vi "Disabled.vi"(7 "Robot Mode":T2, 10 "Match Info":T1={"Autonomous Elapsed Seconds"=0.0, "TeleOp Elapsed Seconds"=0.0, "Disabled Elapsed Seconds"=0.0, "Visited Autonomous"=FALSE, "Visited TeleOp"=FALSE, "Visited Disabled"=FALSE, "Autonomous Settings"={"Autonomous Style"=enum."Independent", "VI Refnum"=refnum}}, 11 "Call Context":T3) -> ()   [LabVIEW 2012]
doc: "This VI is called each time a disabled packet is received from the DS. It is often used to prepare for the next robot mode, to calibrate sensors, etc."
uses:
  <vilib>/Rock Robotics/WPI/DriverStation/WPI_DriverStationDerivedRobotMode.ctl
  <vilib>/Rock Robotics/WPI/DriverStation/WPI_DriverStationRobotMode2.ctl
  <vilib>/Rock Robotics/WPI/DriverStation/WPI_DriverStationMatch Info.ctl
  Robot Global Data.vi
panel:
  out "Boolean Array 2":bool[](array[boolean])
  in  "Boolean Array":bool[](array[boolean])
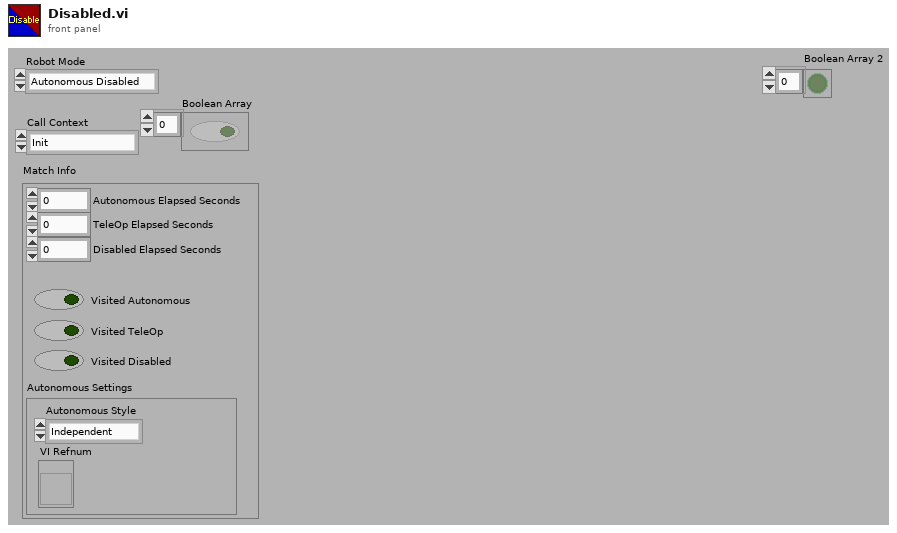
[diagram p1: front panel]
types:
  T1 = typedef "WPI_DriverStationMatch Info.ctl" = cluster{"Autonomous Elapsed Seconds":dbl, "TeleOp Elapsed Seconds":dbl, "Disabled Elapsed Seconds":dbl, "Visited Autonomous":bool, "Visited TeleOp":bool, "Visited Disabled":bool, "Autonomous Settings":cluster{"Autonomous Style":enum16{"Iterative", "Independent"}, "VI Refnum":refnum<vi>}}
  T2 = typedef "WPI_DriverStationRobotMode2.ctl" = enum16{"Autonomous Disabled", "Autonomous Enabled", "Teleop Disabled", "Teleop Enabled", "Timeout", "Finish", "Test Disabled", "Test Enabled"}
  T3 = typedef "WPI_DriverStationDerivedRobotMode.ctl" = enum16{"Init", "Execute", "Stop"}
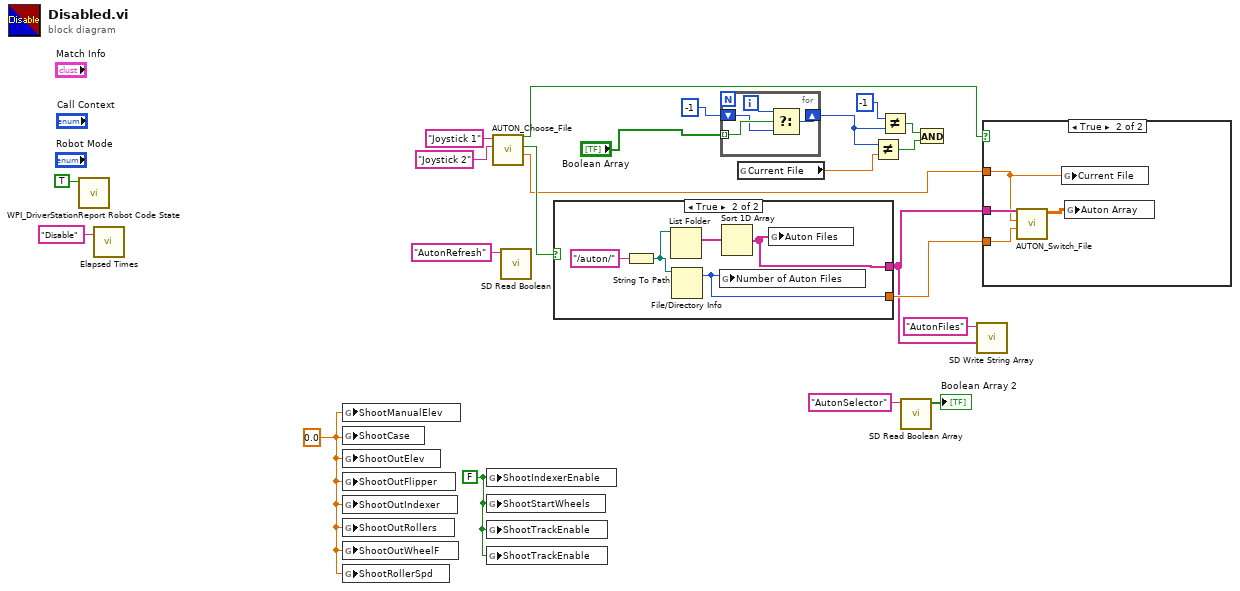
[diagram p0: block diagram]
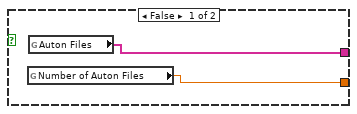
[diagram p3: hidden frame]
diagram:
  w19 = FALSE ("ShootIndexerEnable")
  w18 = 0.0 ("ShootCase")
  n1 = call <vilib>:"WPI_DriverStationReport Robot Code State.vi"("Disabled"=TRUE ("Autonomous")) -> ()  [unwired: 10 in, 1 out]
  n2 = call "Elapsed Times.vi"("Call Name"="Disable") -> ()  [unwired: 2 in, 1 out]
  n3 = global write "Robot Global Data.vi" "ShootManualElev"(w18) -> ()
  n4 = global write "Robot Global Data.vi" "ShootCase"(w18) -> ()
  n5 = global write "Robot Global Data.vi" "ShootOutElev"(w18) -> ()
  n6 = global write "Robot Global Data.vi" "ShootOutFlipper"(w18) -> ()
  n7 = global write "Robot Global Data.vi" "ShootOutIndexer"(w18) -> ()
  n8 = global write "Robot Global Data.vi" "ShootOutRollers"(w18) -> ()
  n9 = global write "Robot Global Data.vi" "ShootOutWheelF"(w18) -> ()
  n10 = global write "Robot Global Data.vi" "ShootRollerSpd"(w18) -> ()
  n11 = global write "Robot Global Data.vi" "ShootIndexerEnable"(w19) -> ()
  n12 = global write "Robot Global Data.vi" "ShootStartWheels"(w19) -> ()
  n13 = global write "Robot Global Data.vi" "ShootTrackEnable"(w19) -> ()
  n14 = global write "Robot Global Data.vi" "ShootTrackEnable"(w19) -> ()
  n15 = call "AUTON_Choose_File.vi"("Joystick 2 Refnum"="Joystick 2" ("Joystick 1 Refnum"), "Joystick 1 Refnum"="Joystick 1") -> ("Auton File"=w3:dbl, "Refresh"=w4:bool, "Allow Change"=w5:bool)  [unwired: 7 in]
  n16 = call <vilib>:"SD Read Boolean.vi"("Name"="AutonRefresh") -> ()  [unwired: 8 in, 3 out]
  n17 = case shown="True" w4 {
    tunnel: [w23 w26] -> w21
    tunnel: [w24 w25] -> w9
    frame False {
      n18 = global read "Robot Global Data.vi" "Number of Auton Files"() -> (w23:dbl)
      n19 = global read "Robot Global Data.vi" "Auton Files"() -> (w24:string[])
    }
    frame True {
      n20 = String To Path(string="/auton/") -> (path=w28:path)
      n21 = List Folder(path=w28) -> (filenames=w27:string[])  [unwired: 3 in, 3 out]
      n22 = File/Directory Info(path=w28) -> (size=w26:i64)  [unwired: 1 in, 6 out]
      n23 = global write "Robot Global Data.vi" "Number of Auton Files"(w26) -> ()
      n24 = Sort 1D Array(array=w27) -> (sorted array=w25:string[])
      n25 = global write "Robot Global Data.vi" "Auton Files"(w25) -> ()
    }
  }
  n26 = for {
    tunnel: "Boolean Array" -> [w33] mode=indexing
    shift-right: [w31] -> w12
    shift-left: -1 -> [w30]
    i -> [w32]
    n27 = Select(t=w32, s=w33, f=w30) -> (s? t:f=w31:i32)
  }
  n28 = global read "Robot Global Data.vi" "Current File"() -> (w15:dbl)
  n29 = Not Equal?(x=w12, y=w15) -> (x != y?=w13:bool)
  n30 = Not Equal?(x=-1, y=w12) -> (x != y?=w14:bool)
  n31 = call <vilib>:"SD Read Boolean Array.vi"("Name"="AutonSelector") -> ("Boolean Array"=→"Boolean Array 2":bool[])  [unwired: 8 in, 2 out]
  n32 = And(x=w14, y=w13) -> ()  [unwired: 1 out]
  n33 = call <vilib>:"SD Write String Array.vi"("String Array"=w9, "Name"="AutonFiles") -> ()  [unwired: 8 in, 2 out]
  n34 = case shown="True" w5 {
    tunnel: w9 -> [_ w37]
    tunnel: w21 -> [_ w36]
    tunnel: w3 -> [_ w34]
    frame False {
    }
    frame True {
      n35 = call "AUTON_Switch_File.vi"("Number of Auton Files"=w36, "Auton File"=w34, "Auton Files"=w37) -> ("Auton Array"=w35:dbl[][])  [unwired: 7 in, 1 out]
      n36 = global write "Robot Global Data.vi" "Current File"(w34) -> ()
      n37 = global write "Robot Global Data.vi" "Auton Array"(w35) -> ()
    }
  }
